vi "Map XML Document.vi"(8 "error in":errorcluster, 11 "XML Document in":refnum<class "XML Document.lvclass">) -> (0 "error out":errorcluster, 3 "XML Document out":refnum<class "XML Document.lvclass">)   [LabVIEW 2014, in "XML Document.lvclass"]
uses:
  XML Document.lvclass
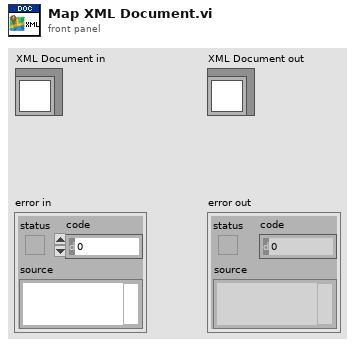
[diagram p1: front panel]
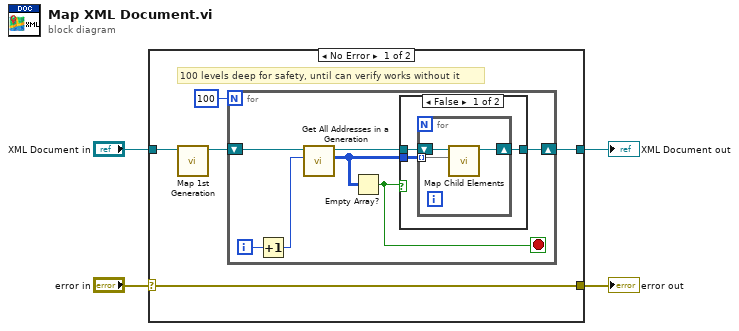
[diagram p0: block diagram]
diagram:
  n1 = case shown="No Error" "error in" {
    selector: "error in" -> [w8 w25]
    tunnel: [w8 w25] -> w3
    tunnel: [w6 w24] -> w1
    tunnel: "XML Document in" -> [w9 w24]
    frame No Error {
      # "100 levels deep for safety, until can verify works without it"
      n2 = call "Map 1st Generation.vi"("XML Document in"=w9) -> ("XML Document out"=w7:refnum<class "XML Document.lvclass">)  [unwired: 9 in, 1 out]
      n3 = for {
        N: 100 -> [_]
        shift-right: [w14] -> w6
        shift-left: w7 -> [w16]
        i -> [w13]
        stop <- w10 stop-if-true
        n4 = Increment(x=w13) -> (x+1=w12:i32)
        n5 = call "Get All Addresses in a Generation.vi"("Generation"=w12, "XML Document in"=w16) -> ("Addresses"=w11:i32[][], "XML Document out"=w15:refnum<class "XML Document.lvclass">)  [unwired: 7 in, 1 out]
        n6 = Empty Array?(array=w11) -> (empty?=w10:bool)
        n7 = case shown="False" w10 {
          tunnel: w15 -> [w19 w23]
          tunnel: [w18 w23] -> w14
          tunnel: w11 -> [w17 _]
          frame False {
            n8 = for {
              shift-right: [w21] -> w18
              shift-left: w19 -> [w22]
              tunnel: w17 -> [w20] mode=indexing
              n9 = call "Map Child Elements.vi"("Address"=w20, "XML Document in"=w22) -> ("XML Document out"=w21:refnum<class "XML Document.lvclass">)  [unwired: 8 in, 1 out]
            }
          }
          frame True {
          }
        }
      }
    }
    frame Error {
    }
  }
  "error out" <- w3
  "XML Document out" <- w1
